vi "Coincidence_rs232(BEREA)WArduino.vi"() -> ()   [LabVIEW 2017]
doc: "This is the program you use to run one of 4 different experiments:\n 1) Simply measuring coincidences between two beams.\n 2) Measuring g(2)(0) for 2-beams using 3-detectors.\n 3) Measuring single photon interference patterns (and simultaneously g(2)(0) for 2-beams using 3-detectors).\n 4) Measuring g(2)(0) for 1-beam using 2-detectors.\nNote that g(2) is calculated differently depending on whether you're making 3-detector or 2-detector measurements. See details in the description of the \"g(2) Measurements\" parameter.\nThis vi was specifically written for the Altera DE2 counter. Data streams to the computer from the DE2 over the RS232 serial port.\nThe program does not record data to a file right away, but displays the counters in real time so that you can align things. \nOnce everything is aligned and the parameters are set, you press the \"Take Data\" button. This transfers control to another program which records a data set and saves it to a file. \nNote that there is one control: \"NewStep?\" that tells the computer what hardware you have present in your experiment. This control is not visible normally. It located below the \"Data Taking Parameters\", so you'll need to scroll the window down to access it. This control is only read once at the beginning of execution--so it must be properly set BEFORE you run the program.\nThe \"NewStep?\" control tells the computer whether or not you have a NewStep stepper motor attached to your computer to control phase adjustments of the interferometer. This control is useful so that the computer won't try to communicate with an instrument you don't have, causing a hang-up. By default \"NewStep?\" is set to \"No\"--if you do have a NewStep, you'll want to change the default to \"Yes\". For more info see the description of this control below.\nFor interference measurements, a Newport NewStep actuator (inexpensive stepper motor) is used to tilt a beam displacing polarizer to adjust the phase of a polarization interferometer. This actuator is controlled by a NewStep controller, connected to a serial port of the computer with an RS-485 to RS-232 converter. If you do not have this controller, set the \"NewStep?\" parameter to \"No\".\nSignals that should be selected on the DE2 for the coincidence counters:\n______________________________________\nA (Counter 0)\nB (Counter 1)\nA' (Counter 2) - unused by this vi\nB' (Counter 3)\nAB (Counter 4)\nABB' (Counter 5) - used for 3-detector g2 measurements (and interference)\nAB' (Counter 6)\nBB' (Counter 7) - used for 2-detector g2 measurements\n__________________________________________________\nNote that for the coincidence experiment, only 3 counters are used: A, B, and AB. For the other 3 experiments, 7 counters are used. \nOn startup, the program initializes the counters.\nAfter initialization the program simply loops and displays the counts in a given time window (determined by the \"Update Period\" control in the upper left.) This is useful for tweaking the alignment and adjusting parameters. \nNothing is written to disk until the parameters are chosen and the \"Take Data\" button is pressed. This loads a second VI that records and saves data to disk. Parameters for this data acquisition phase are set in the \"Data Taking Parameters\" box.\nWhen performing an interference experiment, the stepper motor will automatically adjust the tilt of the beam displacing prism, changing the phase. \nHelp for each of the controls and indicators can be obtained from the Contextual Help window <cntrl - H> by mousing over each control or indicator. Full documentation for each control and indicator can be obtained by printing using: File>Print>Custom, and then checking \"All controls\" and \"Descriptions\"."
uses:
  <vilib>/MakerHub/LINX/Public/Peripherals/Analog/Analog Read 1 Chan.vi
  <vilib>/MakerHub/LINX/Private/Local IO/LinxI2cWrite.vi
  <vilib>/MakerHub/LINX/Public/Utilities/Check Channel.vi
  <vilib>/MakerHub/LINX/Public/Peripherals/Analog/Analog Read N Chans.vi
  <vilib>/MakerHub/LINX/Private/Local IO/LinxAnalogRead.vi
  <vilib>/MakerHub/LINX/Public/Utilities/Open Serial.vi
  <vilib>/MakerHub/LINX/Private/Utilties/Generate Error.vi
  <vilib>/Utility/file.llb/Write Delimited Spreadsheet (DBL).vi
  <vilib>/MakerHub/LINX/LMH-LINX.lvlib
panel:
  out "Current Value of \nDAC  input":u16
  in  "?":T1(tab)
  in  "Tab Control":enum32{"Data Acquisition"}(tab)
  in  "Update Period (Data Run)":dbl=1.0 min=0.1 max=1000.0 step=0.1 format="%.1f"
  in  "Range to scan (±)":u32=100
  in  "Center stepper position\n(µsteps)":u32=26000 min=10000 max=50000 step=1
  in  "Number of points":i32=3
  in  "Take Data":bool
  in  "g(2) Measurements":enum32{"Page 1", "Page 2"}(tab)
  in  "Clear Buffer":bool
  out "Buffer size":u32=60
  out "g(2)":dbl=nan format="%.3f"
  in  "Max Buffer":u32=60
  out "g(2) Std. Dev.":dbl=nan format="%.3f"
  out "Ave.g(2)":dbl=nan format="%.3f"
  in  "Experimental\n Setup":i32(knob) min=0 max=3 step=1 scale=0.0..3.0
  out "Device Name":string
  in  "Counter Port":refnum<visa-resource-name>="COM3"
  in  "Arduino Serial Port":refnum<visa-resource-name>="N/A"
  in  "Update Period":dbl=0.30000000000000004 min=0.1 max=200.0 step=0.1 format="%.1f"
  out "Error Out":errorcluster
  in  "ABB' Coincidence\n window":dbl=4.76 caption="ABB' Coincidence \nWindow (ns)" min=0.1 max=500000.0 step=0.01 format="%.2f"
  in  "2D window stdev":dbl=0.03 caption="+" min=0.0 max=500000.0 step=0.001 format="%.2f"
  in  "BB' Coincidence\n window":dbl=7.39 caption="BB' Coincidence \nWindow (ns)" min=0.1 max=500000.0 step=0.01 format="%.2f"
  in  "Set DAC to 0":bool
  in  "Ramp DAC":bool
  in  "Save Data":bool
  out "Expt ind":i32
  in  "graphs 2":enum32{"B & B'", "BB'", "g(2)(0)"}(tab)
  out "BB'":u32(graph)
  out "g2":dbl(graph)=nan
  out "BB'":u32(slide) scale=0.0..3500.0 scale format="%_2p"
  in  "graphs":T2(tab)
  out "B & B'":cluster{u32, u32}(graph)
  out "AB & AB'":cluster{u32, u32}(graph)
  out "g2":dbl(graph)=nan
  out "BB' vs Voltage":cluster{u32, u32, u32}(graph)
  in  "?":enum32{"Stepper Control"}(tab)
  out "ABB'":u32(slide) scale=0.0..30.0 scale format="%_2p"
  out "B & B'":u32[](array[slide]) scale=0.0..250000.0 scale format="%_2p"
  out "A":u32(slide) scale=0.0..500000.0 scale format="%_2p"
  in  "stop":bool
  out "AB &  AB'":u32[](array[slide]) scale=0.0..20000.0 scale format="%_2p"
  # "AB'"
  # "AB"
  # "B"
  # "B'"
  # "Data Taking Parameters"
  # "(must be a \nmultiple of 0.1s)"
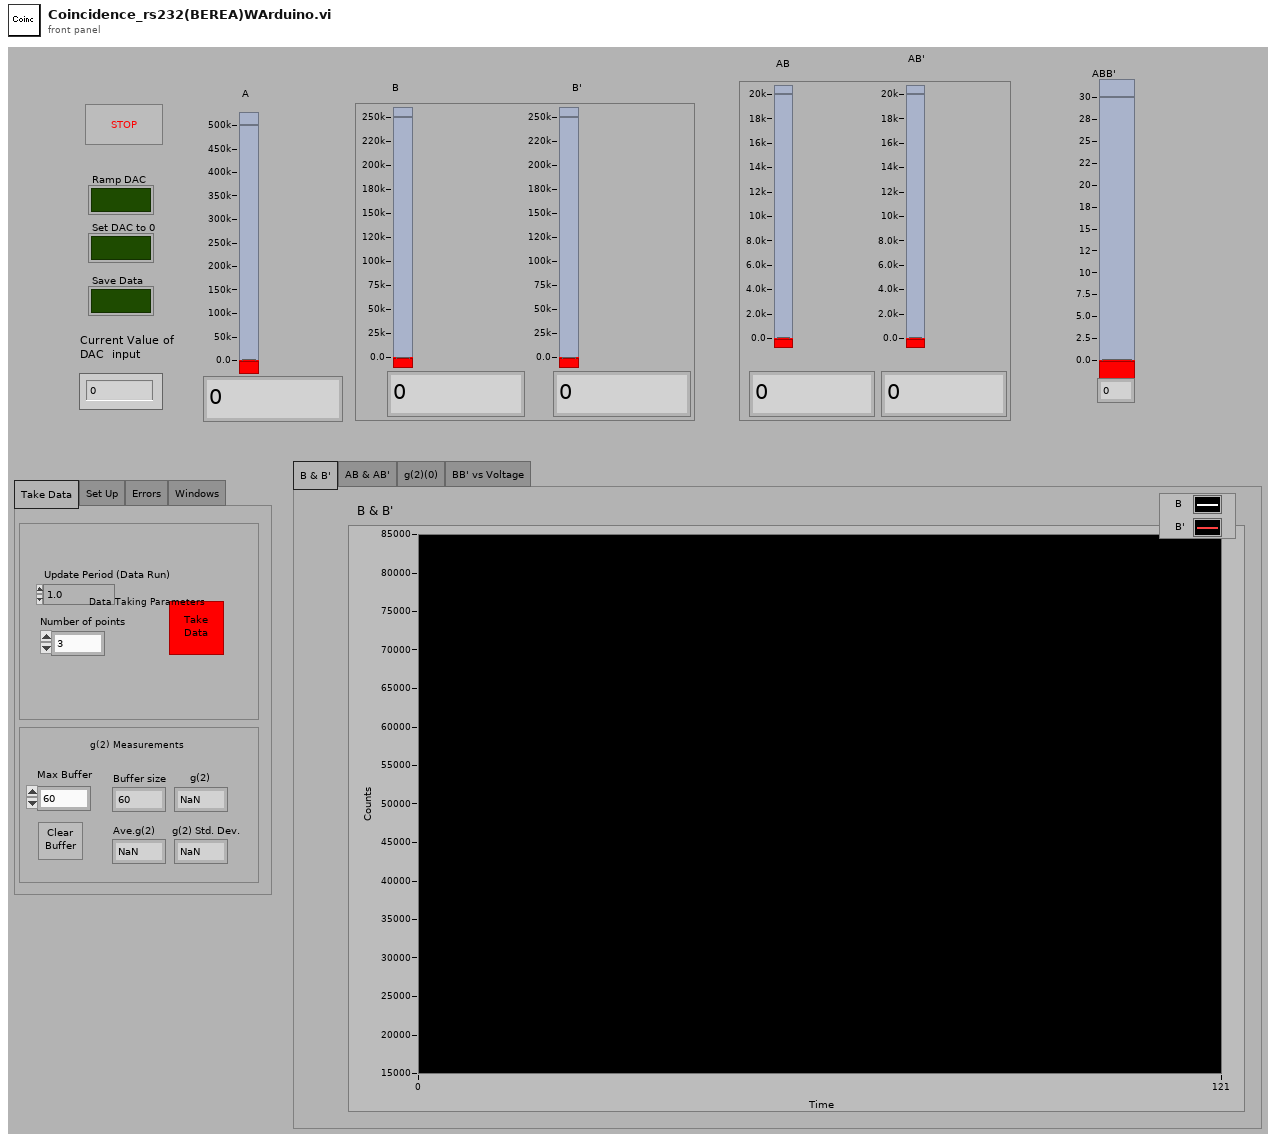
[diagram p1: front panel]
types:
  T1 = enum32{"Take Data", "Set Up", "Errors", "Windows"}
  T2 = enum32{"B & B'", "AB & AB'", "g(2)(0)", "BB' vs Voltage"}
  T3 = typedef "LMH-LINX.lvlib/LINX Ref.ctl" = cluster{"IO":T4, "Interface":T5, "LINX Device Config":T6}
  T4 = typedef "LMH-LINX.lvlib/Platform.ctl" = enum16{"Remote", "Local"}
  T5 = typedef "LMH-LINX.lvlib/Interface.ctl" = enum16{"Serial", "TCP"}
  T6 = typedef "LMH-LINX.lvlib/Device.lvlib/LINX Device Config.ctl" = cluster{"Interface":T5, "COM Port":refnum<visa-resource-name>, "TCP Configuration":T7, "Device Family":u8, "Device ID":u8, "Device Name":string, "TCP Ref":refnum<k5>, "Channels":T8}
  T7 = typedef "LMH-LINX.lvlib/Device.lvlib/TCP Config.ctl" = cluster{"IP Address":string, "Port":u16}
  T8 = typedef "LMH-LINX.lvlib/Channels.ctl" = cluster{"DI":u8[], "DO":u8[], "AI":u8[], "AO":u8[], "PWM":u8[], "QE":u8[], "UART":u8[], "I2C 2":u8[], "SPI":u8[], "CAN":u8[], "Servo":u8[], "AI Ref (V)":dbl, "AI Resolution (Bits)":u8, "AO Ref (V)":dbl, "AO Resolution (Bits)":u8}
  T9 = cluster{"BB' Coincidence\n window":dbl, "2D window stdev":dbl, "ABB' Coincidence\n window":dbl}
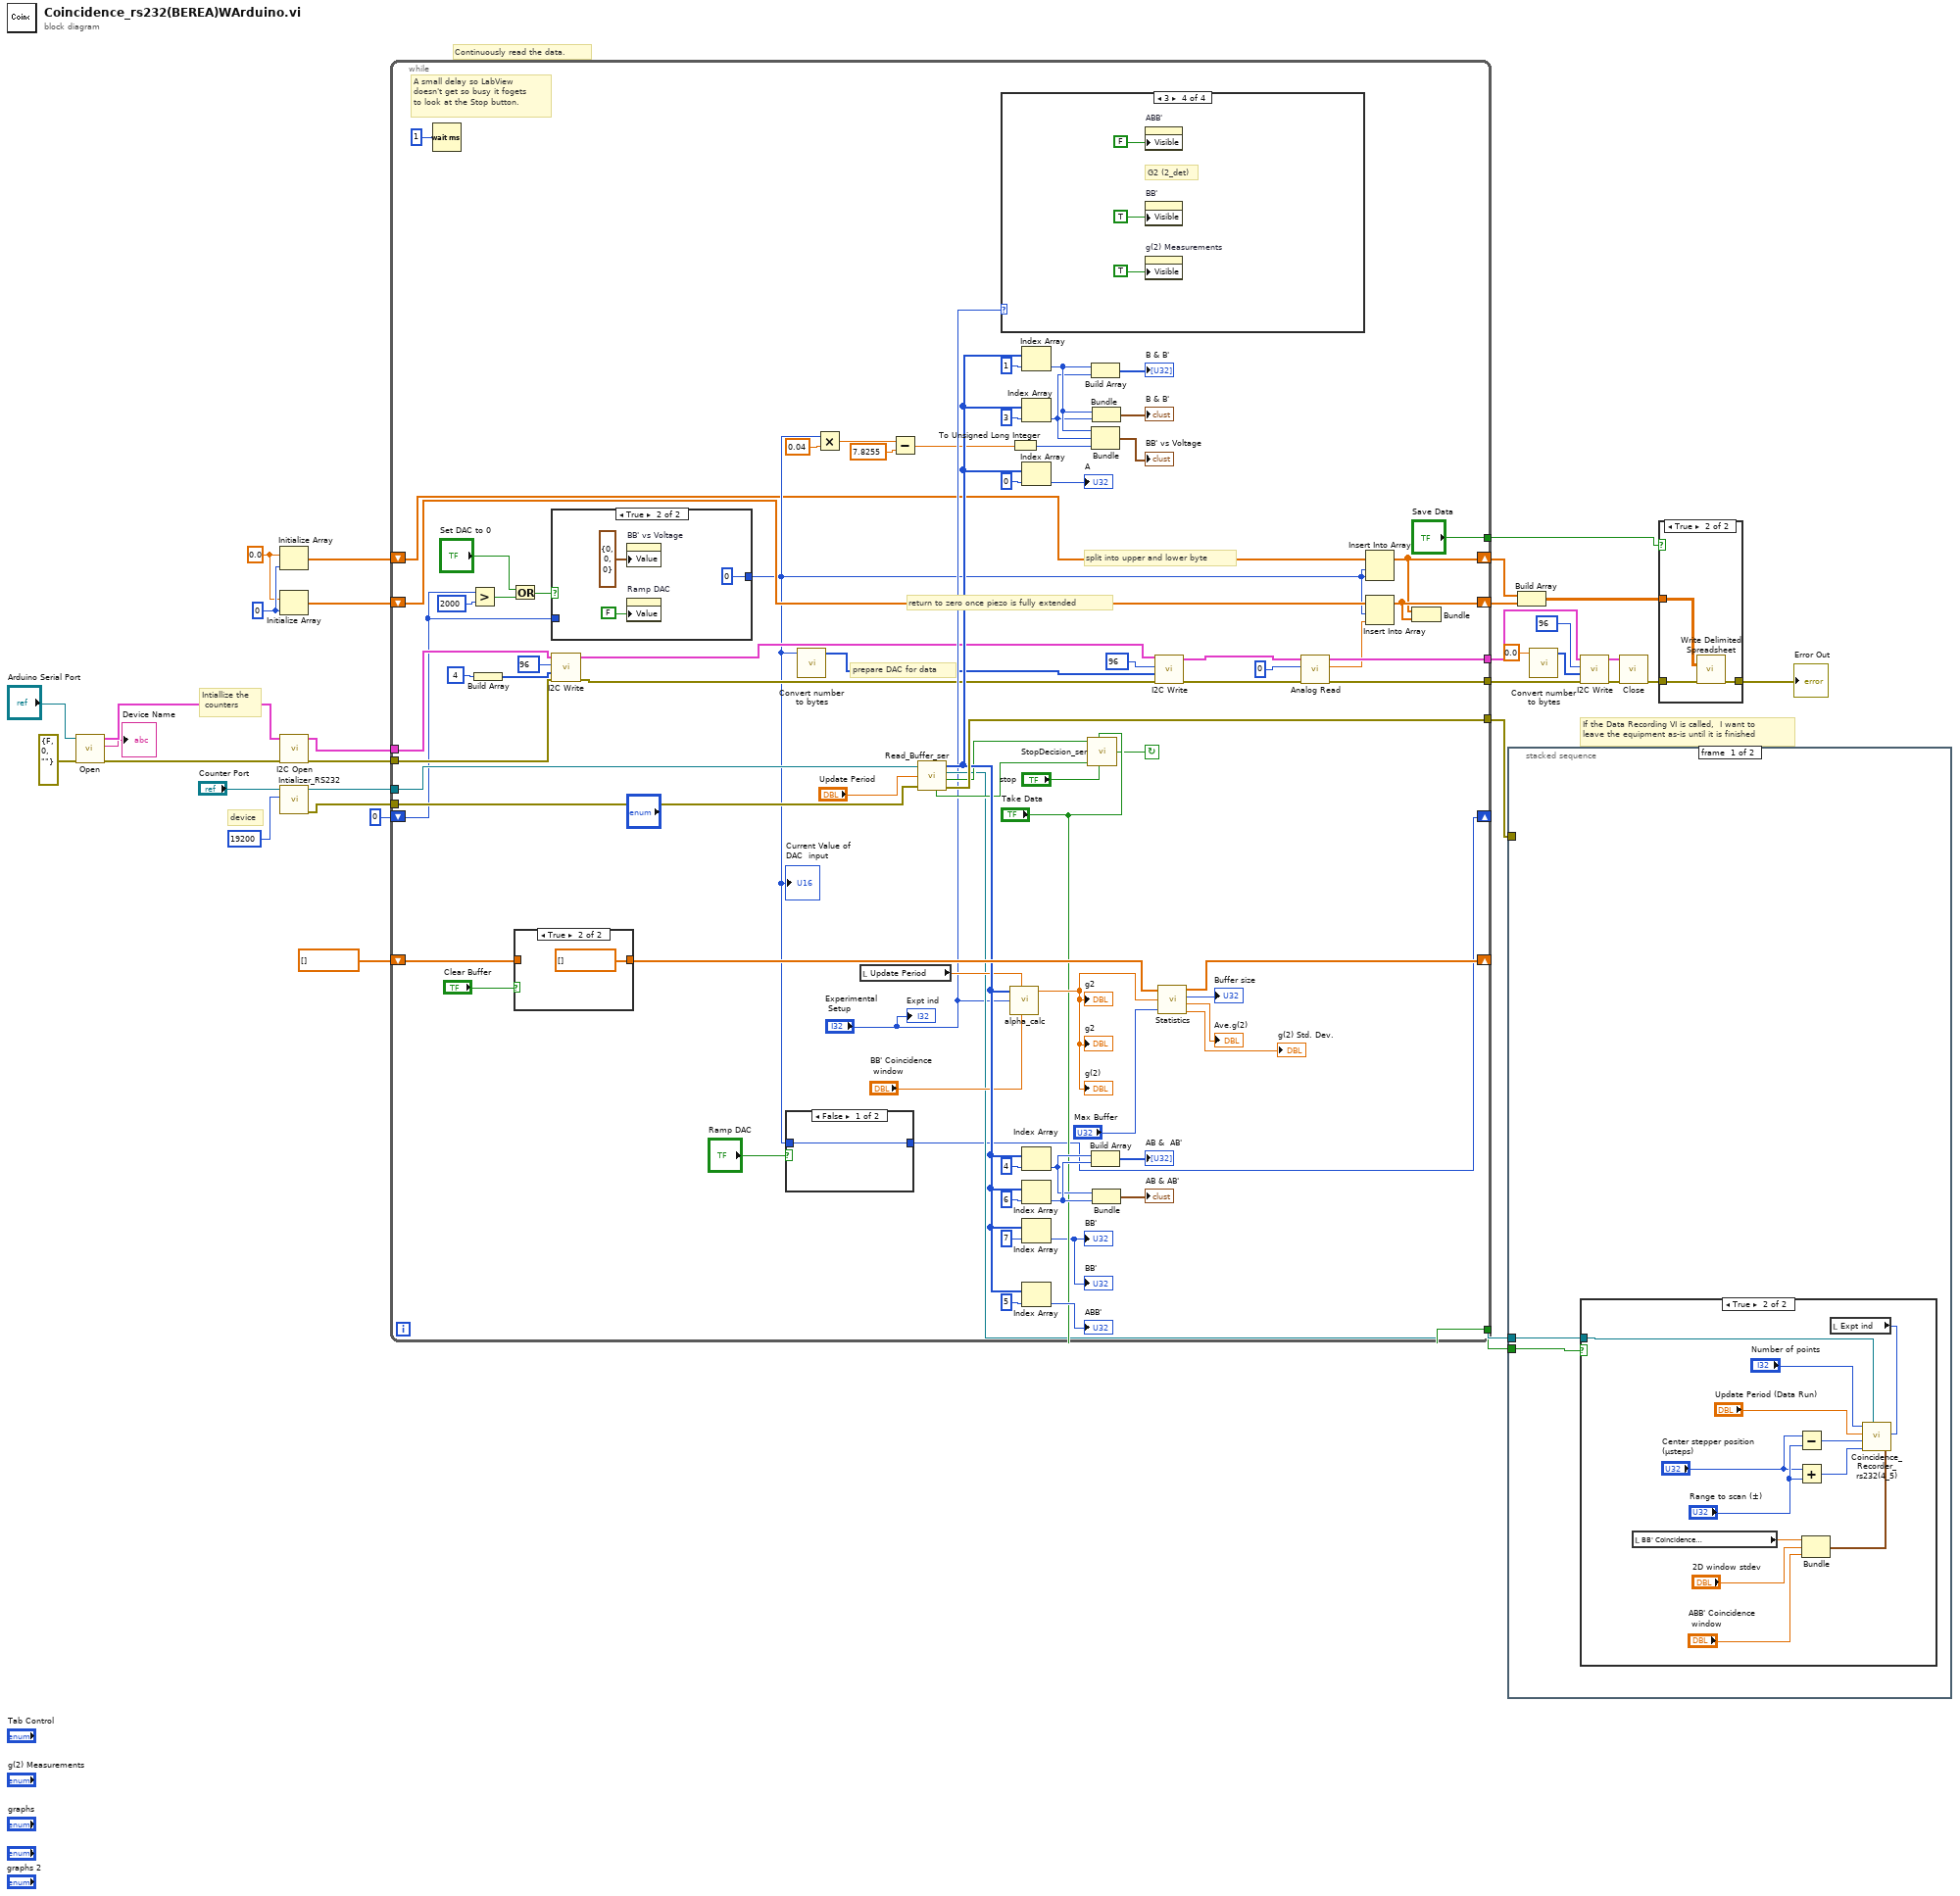
[diagram p0: block diagram]
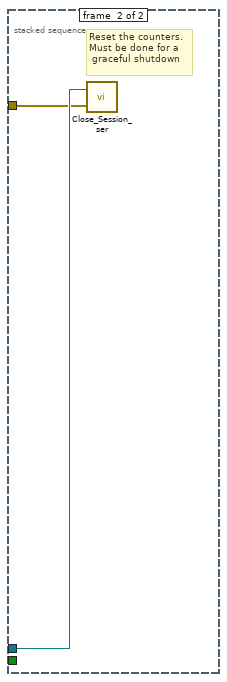
[diagram p4: hidden frame]
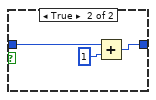
[diagram p5: hidden frame]
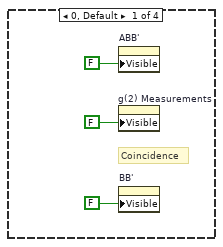
[diagram p8: hidden frame]
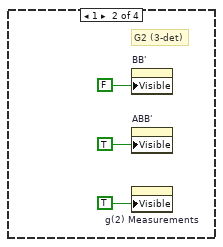
[diagram p9: hidden frame]
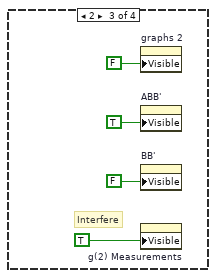
[diagram p10: hidden frame]
diagram:
  w14 = 0.0 ("element")
  w15 = 0 ("dimension size")
  # "If the Data Recording VI is called,  I want to \nleave the equipment as-is until it is finished"
  # "Intiallize the\n counters"
  # "Continuously read the data."
  # "device"
  n1 = call-poly <vilib>:"Open.vi"("Error In"=errorcluster {"status"=FALSE, "code"=0, "source"=""}, "Serial Port"="Arduino Serial Port") -> ("Error Out"=w23:errorcluster, "Device Name"=→"Device Name":string, "LINX Resource"=w24:T3)  [unwired: 7 in]
  n2 = Initialize Array(w14, w15) -> (w8:dbl[])
  n3 = Initialize Array(w14, w15) -> (w7:dbl[])
  n4 = call <vilib>:"I2C Open.vi"("Error In"=w23, "LINX Resource"=w24) -> ("Error Out"=w9:errorcluster, "LINX Resource"=w10:T3)  [unwired: 8 in]
  n5 = call "Intializer_RS232.vi"("baud rate"=u32 19200 ("device"), "Counter Port"="Counter Port") -> ("error out"=w32:errorcluster, "Counter port out"=w31:refnum<visa-resource-name>)  [unwired: 4 in]
  n6 = while {
    tunnel: w31 -> [w73]
    tunnel: w32 -> [w105]
    tunnel: [w104] -> w27
    tunnel: [w72] -> w29
    shift-right: [w90] -> _
    shift-left: dbl[] [] ("Output Array") -> [w92]
    tunnel: ["Take Data"] -> w28
    tunnel: w10 -> [w52]
    tunnel: w9 -> [w51]
    tunnel: [w69] -> w2
    tunnel: ["Save Data"] -> w4
    shift-right: [w53] -> _
    shift-left: 0 -> [w50]
    tunnel: [w48] -> w1
    shift-right: [w47] -> w5
    shift-left: w7 -> [w70]
    shift-right: [w46] -> w6
    shift-left: w8 -> [w49]
    stop <- w75 continue-if-true
    # "prepare DAC for data"
    # "return to zero once piezo is fully extended"
    # "split into upper and lower byte"
    # "A small delay so LabView\ndoesn't get so busy it fogets\nto look at the Stop button."
    n7 = Wait (ms)(milliseconds to wait=u32 1) -> ()  [unwired: 1 out]
    n8 = Greater?(x=w50, y=2000) -> (0:w43:bool)
    n9 = Build Array(u8 4) -> (w64:u8[])
    n10 = Or(x="Set DAC to 0", y=w43) -> (x .or. y?=w42:bool)
    n11 = case shown="True" "Clear Buffer" {
      tunnel: w92 -> [w118 _]
      tunnel: [w118 dbl[] [] ("Output Array")] -> w91
      frame False {
      }
      frame True {
      }
    }
    n12 = case shown="True" w42 {
      tunnel: [w114 0] -> w55
      tunnel: w50 -> [w114 _]
      frame False {
      }
      frame True {
        n13 = property on="BB' vs Voltage" class="WFChart (strict)"("Value"=cluster{u32, u32, u32} {0, 0, 0} ("BB' vs Voltage")) -> ()  [unwired: 2 in, 2 out]
        n14 = property on="Ramp DAC" class="Bool (strict)"("Value"=FALSE ("Boolean")) -> ()  [unwired: 2 in, 2 out]
      }
    }
    "Current Value of \nDAC  input" <- w55
    n15 = call <vilib>:"I2C Write.vi"("Error In"=w51, "Data"=w64, "I2C Slave Address (0)"=u8 96, "LINX Resource"=w52) -> ("Error Out"=w60:errorcluster, "LINX Resource"=w59:T3)  [unwired: 6 in]
    n16 = case shown="False" "Ramp DAC" {
      tunnel: w55 -> [w110 w112]
      tunnel: [w110 w111] -> w53
      frame False {
      }
      frame True {
        n17 = Add(x=w112, y=1) -> (x+y=w111:i32)
      }
    }
    n18 = call "Convert number to bytes.vi"("Numeric"=w55) -> ("Array"=w68:u8[])  [unwired: 10 in]
    n19 = Multiply(x=w55, y=0.04) -> (x*y=w58:dbl)
    n20 = local read "Update Period"() -> (w80:dbl)
    n21 = Subtract(x=w58, y=7.8255) -> (x-y=w38:dbl)
    n22 = call "Read_Buffer_ser.vi"("error in"=w105, "Update Period (s)"="Update Period", "Counter Port"=w73) -> ("error out"=w104:errorcluster, "status"=w78:bool, "Finished"=w79:bool, "Counter port out"=w72:refnum<visa-resource-name>, "The actual numbers"=w82:u32[])  [unwired: 1 in]
    n23 = case shown="3" "Experimental\n Setup" {
      frame 0, Default {
        # "Coincidence"
        n24 = property on="ABB'" class="Slide (strict)"("Visible"=FALSE) -> ()  [unwired: 2 in, 2 out]
        n25 = property on="g(2) Measurements" class="TabCtl (strict)"("Visible"=FALSE) -> ()  [unwired: 2 in, 2 out]
        n26 = property on="BB'" class="Slide (strict)"("Visible"=FALSE) -> ()  [unwired: 2 in, 2 out]
      }
      frame 1 {
        # "G2 (3-det)"
        n27 = property on="BB'" class="Slide (strict)"("Visible"=FALSE) -> ()  [unwired: 2 in, 2 out]
        n28 = property on="ABB'" class="Slide (strict)"("Visible"=TRUE) -> ()  [unwired: 2 in, 2 out]
        n29 = property on="g(2) Measurements" class="TabCtl (strict)"("Visible"=TRUE) -> ()  [unwired: 2 in, 2 out]
      }
      frame 2 {
        # "Interfere"
        n30 = property on="graphs 2" class="TabCtl (strict)"("Visible"=FALSE) -> ()  [unwired: 2 in, 2 out]
        n31 = property on="ABB'" class="Slide (strict)"("Visible"=TRUE) -> ()  [unwired: 2 in, 2 out]
        n32 = property on="BB'" class="Slide (strict)"("Visible"=FALSE) -> ()  [unwired: 2 in, 2 out]
        n33 = property on="g(2) Measurements" class="TabCtl (strict)"("Visible"=TRUE) -> ()  [unwired: 2 in, 2 out]
      }
      frame 3 {
        # "G2 (2_det)"
        n34 = property on="ABB'" class="Slide (strict)"("Visible"=FALSE) -> ()  [unwired: 2 in, 2 out]
        n35 = property on="BB'" class="Slide (strict)"("Visible"=TRUE) -> ()  [unwired: 2 in, 2 out]
        n36 = property on="g(2) Measurements" class="TabCtl (strict)"("Visible"=TRUE) -> ()  [unwired: 2 in, 2 out]
      }
    }
    n37 = call "alpha_calc.vi"("data"=w82, "Update Period"=w80, "Experiment"="Experimental\n Setup", "Coincidence\n window"="BB' Coincidence\n window") -> ("Alpha"=w83:dbl)  [unwired: 3 in]
    "g(2)" <- w83
    "g2" <- w83
    "g2" <- w83
    n38 = To Unsigned Long Integer(number=w38) -> (unsigned 32bit integer=w37:u32)
    n39 = Index Array(array=w82, index=1) -> (element=w35:u32)
    n40 = Index Array(array=w82, index=3) -> (element=w34:u32)
    n41 = Index Array(array=w82, index=0) -> (element=→"A":u32)
    n42 = Index Array(array=w82, index=4) -> (element=w95:u32)
    n43 = Index Array(array=w82, index=6) -> (element=w96:u32)
    n44 = Index Array(array=w82, index=7) -> (element=→"BB'" →"BB'":u32)
    n45 = Index Array(array=w82, index=5) -> (element=→"ABB'":u32)
    n46 = call "StopDecision_ser.vi"("Stop Button"="stop", "Take Data Button"="Take Data", "STATUS"=w78, "Finished? 1"=w79) -> ("To \"Continue if true\""=w75:bool)  [unwired: 2 in]
    n47 = Build Array(w35, w34) -> (→"B & B'":u32[])
    n48 = Bundle(w35, w34, w37) -> (→"BB' vs Voltage":cluster{u32, u32, u32})  [unwired: 1 in]
    n49 = Build Array(w95, w96) -> (→"AB &  AB'":u32[])
    n50 = Bundle(w35, w34) -> (→"B & B'":cluster{u32, u32})  [unwired: 1 in]
    n51 = Bundle(w95, w96) -> (→"AB & AB'":cluster{u32, u32})  [unwired: 1 in]
    n52 = call <vilib>:"I2C Write.vi"("Error In"=w60, "Data"=w68, "I2C Slave Address (0)"=u8 96, "LINX Resource"=w59) -> ("Error Out"=w62:errorcluster, "LINX Resource"=w63:T3)  [unwired: 6 in]
    n53 = call "Statistics.vi"("Input Array"=w91, "Array element"=w83, "Max. Array Size"="Max Buffer") -> ("Output Array"=w90:dbl[], "Array size"=→"Buffer size":u32, "Mean"=→"Ave.g(2)":dbl, "Std. Dev."=→"g(2) Std. Dev.":dbl)
    n54 = call-poly <vilib>:"Analog Read.vi"("Error In"=w62, "Analog Channel"=u8 0, "LINX Resource"=w63) -> ("Error Out"=w48:errorcluster, "Voltage"=w40:dbl, "LINX Resource"=w69:T3)  [unwired: 5 in, 1 out]
    n55 = Insert Into Array(array=w49, index=w55, new element=w55) -> (w46:dbl[])
    n56 = Insert Into Array(array=w70, index=w55, new element=w40) -> (w47:dbl[])
    n57 = Bundle(w46, w47) -> ()  [unwired: 1 in, 1 out]
    "Expt ind" <- "Experimental\n Setup"
  }
  n58 = stacked-sequence {
    tunnel: w29 -> [w134 w148]
    tunnel: w28 -> [w133 _]
    tunnel: w27 -> [_ w147]
    frame #0 {
      n59 = case shown="True" w133 {
        tunnel: w134 -> [_ w144]
        frame False {
        }
        frame True {
          n60 = local read "BB' Coincidence\n window"() -> (w138:dbl)
          n61 = Subtract(x="Center stepper position\n(µsteps)", y="Range to scan (±)") -> (x-y=w143:u32)
          n62 = Add(x="Center stepper position\n(µsteps)", y="Range to scan (±)") -> (x+y=w142:u32)
          n63 = Bundle("BB' Coincidence\n window"=w138, "2D window stdev"="2D window stdev", "ABB' Coincidence\n window"="ABB' Coincidence\n window") -> (w137:T9)  [unwired: 1 in]
          n64 = local read "Expt ind"() -> (w139:i32)
          n65 = call "Coincidence_Recorder_rs232(4_5).vi"("Coincidence times"=w137, "Experiment"=w139, "Counter Port"=w144, "End stepper position"=w142, "Starting stepper position"=w143, "Time per update (s)"="Update Period (Data Run)", "Number of points"="Number of points") -> ()  [unwired: 3 in]
        }
      }
    }
    frame #1 {
      # "Reset the counters.\nMust be done for a\n graceful shutdown"
      n66 = call "Close_Session_ser.vi"("error in (no error)"=w147, "Counter Port"=w148) -> ()  [unwired: 1 in]
    }
  }
  n67 = Build Array(w6, w5) -> (w11:dbl[][])
  n68 = call "Convert number to bytes.vi"("Numeric"=0.0) -> ("Array"=w19:u8[])  [unwired: 10 in]
  n69 = call <vilib>:"I2C Write.vi"("Error In"=w1, "Data"=w19, "I2C Slave Address (0)"=u8 96, "LINX Resource"=w2) -> ("Error Out"=w18:errorcluster, "LINX Resource"=w17:T3)  [unwired: 6 in]
  n70 = call <vilib>:"Close.vi"("Error In"=w18, "LINX Resource"=w17) -> ("Error Out"=w13:errorcluster)  [unwired: 9 in]
  n71 = case shown="True" w4 {
    tunnel: [w149 w152] -> w12
    tunnel: w13 -> [w149 w150]
    tunnel: w11 -> [_ w151]
    frame False {
    }
    frame True {
      n72 = call-poly <vilib>:"Write Delimited Spreadsheet.vi"("2D data"=w151, "error in (no error)"=w150) -> ("error out"=w152:errorcluster)  [unwired: 12 in, 1 out]
    }
  }
  "Error Out" <- w12
